vi "Get Joystick State.vi"(8 "error in (no error)":errorcluster, 11 "RPI.SenseHat.Actor in":refnum<class "RPI.SenseHat.Actor.lvclass">) -> (0 "error out":errorcluster, 3 "RPI.SenseHat.Actor out":refnum<class "RPI.SenseHat.Actor.lvclass">)   [LabVIEW 2020, in "RPI.SenseHat.Actor.lvlib" / "RPI.SenseHat.Actor.lvclass"]
uses:
  RPI.SenseHat.Actor.lvclass
  RPI.SenseHat.Actor.lvclass/RPI.SenseHat.Actor.ctl
  RPI.SenseHat/SenseHat/SenseHat.lvclass/SenseHat.ctl
  RPI.SenseHat/SenseHat/Get RPI.SenseHat.Joystick.vi
  RPI.SenseHat.Joystick/Classes/senseHatJoystick/RPI.SenseHat.Joystick.lvclass
  RPI.SenseHat/SenseHat/SenseHat.lvclass
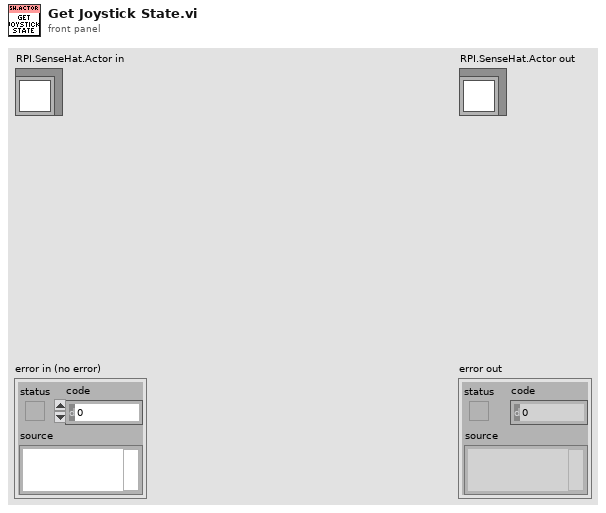
[diagram p1: front panel]
types:
  T1 = typedef "RPI.SenseHat.Joystick.lvlib/Joystick.ctl" = cluster{"Enter":bool, "Down":bool, "Up":bool, "Right":bool, "Left":bool}
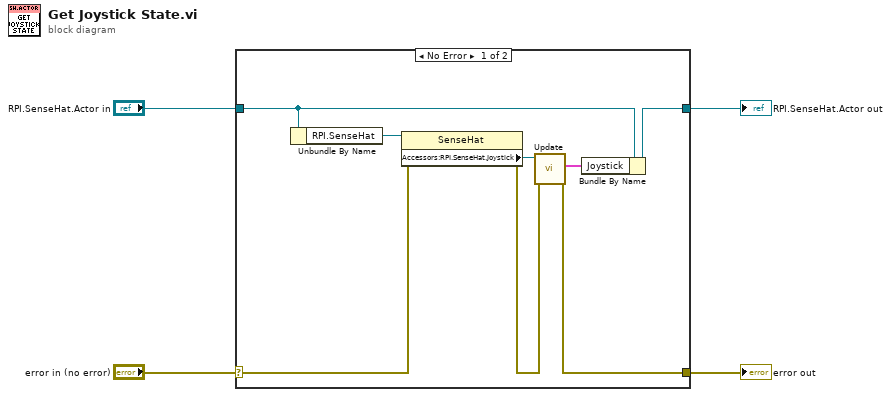
[diagram p0: block diagram]
diagram:
  n1 = case shown="No Error" "error in (no error)" {
    selector: "error in (no error)" -> [w9 w14]
    tunnel: [w8 w14] -> w3
    tunnel: [w5 w13] -> w1
    tunnel: "RPI.SenseHat.Actor in" -> [w7 w13]
    frame No Error {
      n2 = Unbundle By Name(w7) -> ("RPI.SenseHat"=w12:refnum<class "SenseHat.lvclass">)
      n3 = property class="SenseHat"(reference=w12, error in=w9) -> (error out=w10:errorcluster, "Accessors:RPI.SenseHat.Joystick"=w11:refnum<class "RPI.SenseHat.Joystick.lvclass">)  [unwired: 1 out]
      n4 = call "Update.vi"("error in (no error)"=w10, "senseHatJoystick in"=w11) -> ("error out"=w8:errorcluster, "Joystick"=w6:T1)  [unwired: 7 in, 1 out]
      n5 = Bundle By Name(cluster=w7, "Joystick"=w6) -> (w5:refnum<class "RPI.SenseHat.Actor.lvclass">)
    }
    frame Error {
    }
  }
  "error out" <- w3
  "RPI.SenseHat.Actor out" <- w1
